vi "Unwrap UDP Payload.vi"(8 "error in (no error)":errorcluster, 9 "Expected Type (Any)":u32, 10 "UDP Payload":string) -> (0 "error out":errorcluster, 2 "Data":T1)   [LabVIEW 2020, in "Vecto.lvlib"]
uses:
  Vecto.lvlib
  proto/UdpPayload/Data.ctl
  proto/UdpPayload/UdpPayload.lvlib
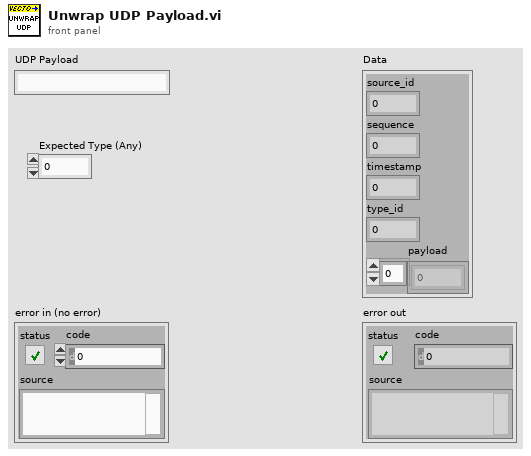
[diagram p1: front panel]
types:
  T1 = typedef "UdpPayload.lvlib/Data.ctl" = cluster{"source_id":u32, "sequence":u32, "timestamp":u64, "type_id":u32, "payload":u8[]}
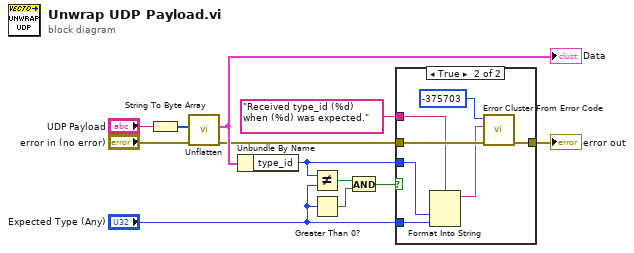
[diagram p0: block diagram]
diagram:
  n1 = String To Byte Array(string="UDP Payload") -> (unsigned byte array=w11:u8[])
  n2 = call "Unflatten.vi"("error in"="error in (no error)", "Buffer"=w11) -> ("error out"=w5:errorcluster, "Data"=w9:T1)  [unwired: 8 in]
  "Data" <- w9
  n3 = Unbundle By Name(w9) -> ("type_id"=w2:u32)
  n4 = Not Equal?(x=w2, y="Expected Type (Any)") -> (x != y?=w8:bool)
  n5 = Greater Than 0?(x="Expected Type (Any)") -> (x > 0?=w7:bool)
  n6 = And(x=w8, y=w7) -> (x .and. y?=w6:bool)
  n7 = case shown="True" w6 {
    tunnel: w5 -> [w13 w20]
    tunnel: [w13 w19] -> w4
    tunnel: "Expected Type (Any)" -> [_ w16]
    tunnel: w2 -> [_ w15]
    tunnel: "Received type_id (%d) when (%d) was expected." -> [_ w17]
    frame False {
    }
    frame True {
      n8 = Format Into String(format string=w17, w15, w16) -> (resulting string=w14:string)  [unwired: 2 in, 1 out]
      n9 = call <vilib>:"Error Cluster From Error Code.vi"("error in (no error)"=w20, "error message (\"\")"=w14, "error code (0)"=-375703) -> ("error out"=w19:errorcluster)  [unwired: 6 in]
    }
  }
  "error out" <- w4
